vi "ServoMotorDriver.vi"() -> ()   [LabVIEW 2022 SP3]
uses:
  <vilib>/DAQmx/write.llb/DAQmx Write (Digital Bool 1Line 1Point).vi
  <vilib>/DAQmx/create/channels.llb/DAQmx Create Channel (DO-Digital Output).vi
  <vilib>/DAQmx/miscellaneous.llb/DAQmx Fill In Error Info.vi
  <vilib>/DAQmx/create/channels.llb/DAQmx Create Channel (CO-Pulse Generation-Frequency).vi
panel:
  in  "milliseconds to wait":u32
  in  "stop":bool
  out "Boolean 2":bool
  in  "lines":tag
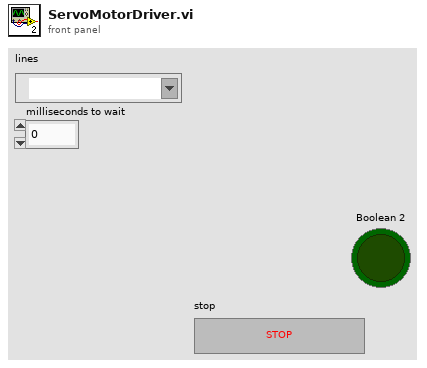
[diagram p1: front panel]
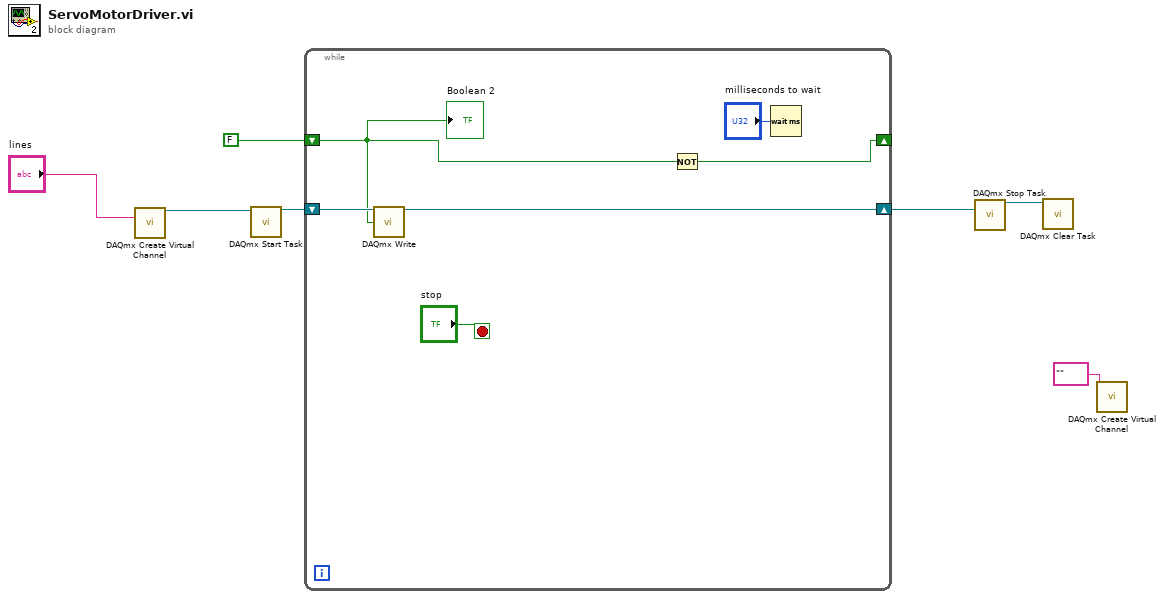
[diagram p0: block diagram]
diagram:
  n1 = call-poly <vilib>:"DAQmx Create Virtual Channel.vi"("lines"="lines") -> ("task out"=w6:refnum<k21>)  [unwired: 13 in, 1 out]
  n2 = call <vilib>:"DAQmx Start Task.vi"("task/channels in"=w6) -> ("task out"=w5:refnum<k21>)  [unwired: 13 in, 1 out]
  n3 = while {
    shift-right: [w12] -> w4
    shift-left: w5 -> [w13]
    shift-right: [w8] -> _
    shift-left: FALSE -> [w9]
    stop <- "stop" stop-if-true
    n4 = call-poly <vilib>:"DAQmx Write.vi"("task/channels in"=w13, "data"=w9) -> ("task out"=w12:refnum<k21>)  [unwired: 11 in, 2 out]
    n5 = Not(x=w9) -> (.not. x?=w8:bool)
    n6 = Wait (ms)(milliseconds to wait="milliseconds to wait") -> ()  [unwired: 1 out]
    "Boolean 2" <- w9
  }
  n7 = call <vilib>:"DAQmx Stop Task.vi"("task/channels in"=w4) -> ("task out"=w3:refnum<k21>)  [unwired: 13 in, 1 out]
  n8 = call <vilib>:"DAQmx Clear Task.vi"("task in"=w3) -> ()  [unwired: 14 in, 1 out]
  n9 = call-poly <vilib>:"DAQmx Create Virtual Channel.vi"("counter"=tag "") -> ()  [unwired: 13 in, 2 out]
